vi "skil4.vi"() -> ()   [LabVIEW 2010]
uses:
  <vilib>/Utility/miscctls.llb/LVRectTypeDef.ctl
  lib/Global 2.vi
  <vilib>/Platform/browser.llb/Open URL in Default Browser (path).vi
panel:
  in  "View":bool
  out "Table":string[][](table)
  out "Dev_Gr":cluster{"DevNo":i32, "Group":string}[](array[cluster])
  out "Horizontal:Memory Size":i32 format="%.0p"
  in  "Ed 2":bool
  in  "Ed":bool
  in  "tm":bool
  out "User":string
  out "Device:Temperature":dbl format="%#4.0f"
  out "GPS:Status":i32(ring) items=["Uninitialized", "Antenna Error", "No Useable Satellites", "One Useable Satellite", "Two Useable Satellites", "Three Useable Satellites", "No GPS Time", "PDOP Too High", "Unuseable Satellite", "Fix Rejected", "Self Survey Complete", "Self Survey Not Complete"]
  out "d_h_m_s":dbl caption="в работе (дни, часы, минуты, секунды)" format="%<%D:%H:%M:%S>t"
  out "# elements in queue":i32 caption="Буфер"
  in  "indexhtm":bool
  in  "stop 2":bool
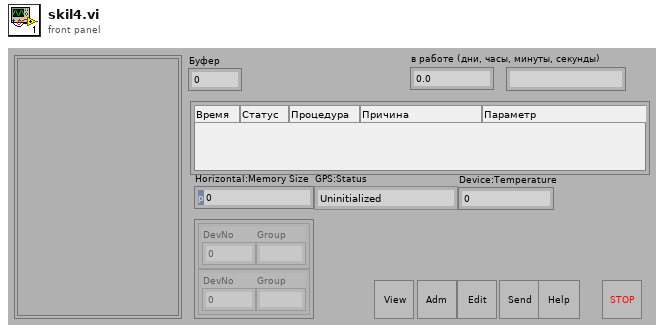
[diagram p1: front panel]
types:
  T1 = cluster{"seconds since 1Jan1904":timestamp, "error out":errorcluster}
  T2 = typedef "LVRectTypeDef.ctl" = cluster{"Left":i16, "Top":i16, "Right":i16, "Bottom":i16}
  T3 = cluster{cluster{"actualSamples":i32, "absoluteInitialX":dbl, "relativeInitialX":dbl, "xIncrement":dbl, "offset":dbl, "gain":dbl, "reserved1":dbl, "reserved2":dbl}[], "wfm":i16[][]}
  T4 = cluster{"Time Stamp":timestamp, "error out":errorcluster}
  T5 = cluster{"adc handle":refnum<k15>, "PN":string, "KR":string}
  T6 = cluster{"seconds since 1Jan1904":timestamp, "error out":errorcluster}[]
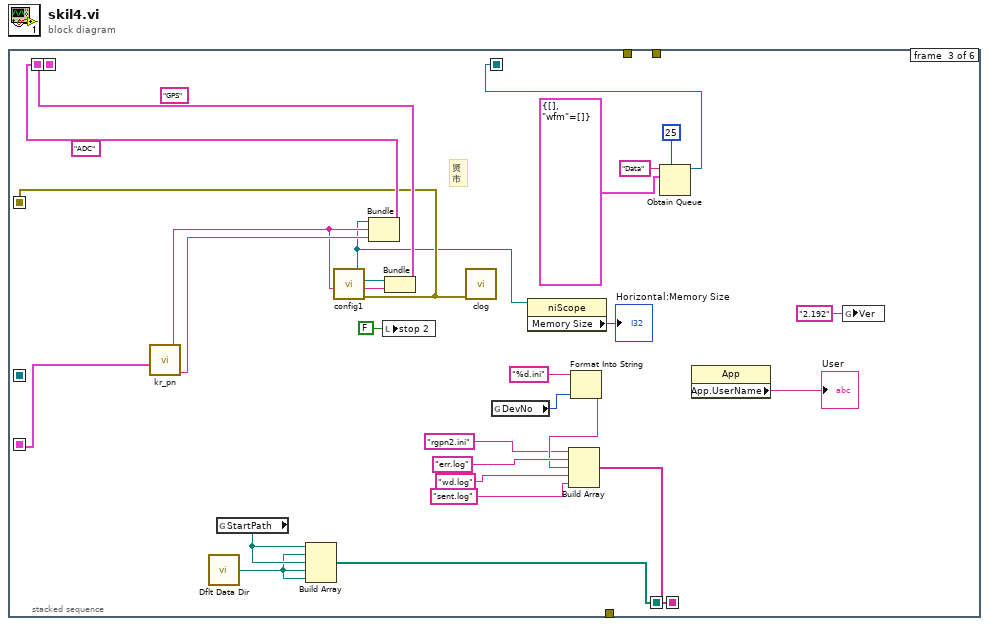
[diagram p0: block diagram]
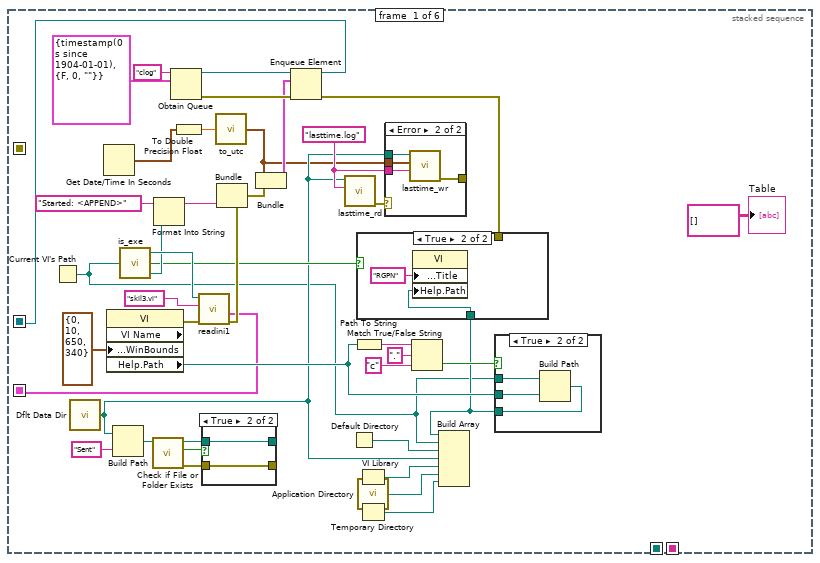
[diagram p2: hidden frame]
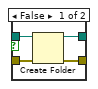
[diagram p6: hidden frame]
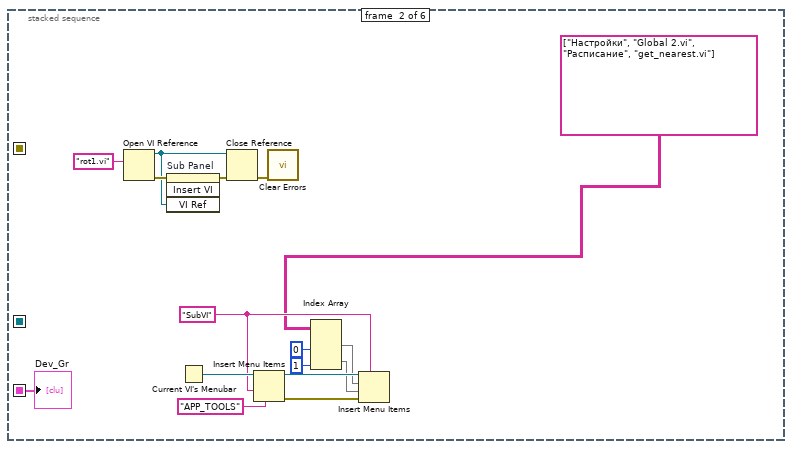
[diagram p7: hidden frame]
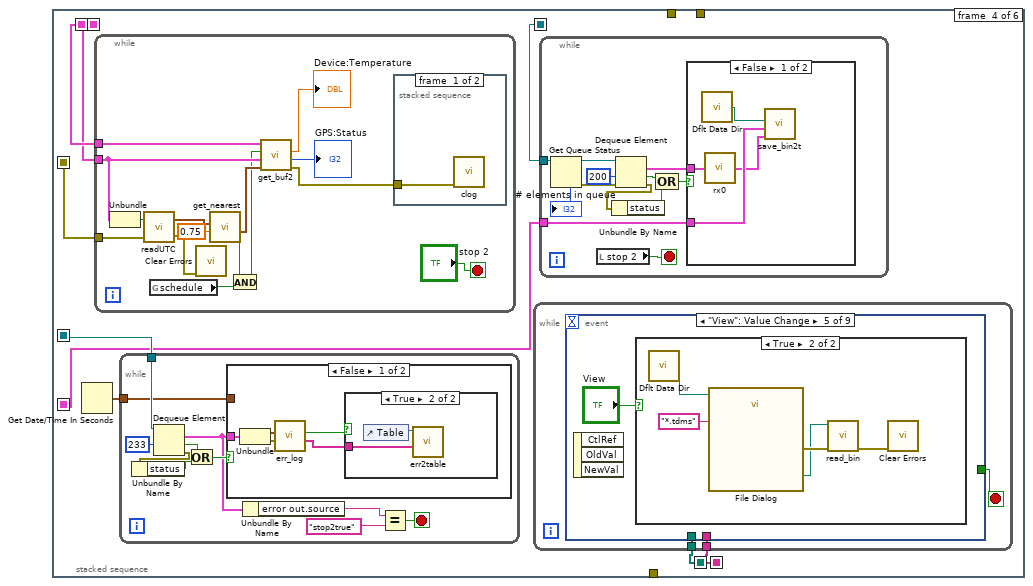
[diagram p8: hidden frame]
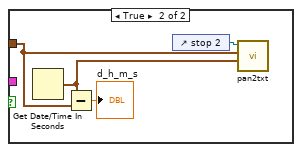
[diagram p10: hidden frame]
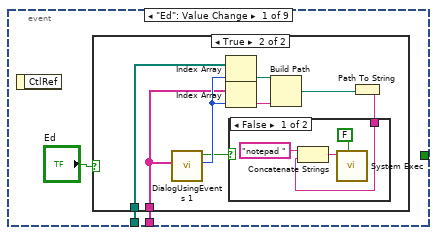
[diagram p11: hidden frame]
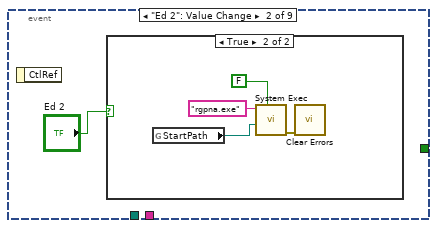
[diagram p14: hidden frame]
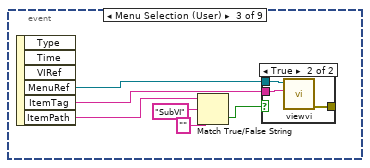
[diagram p16: hidden frame]
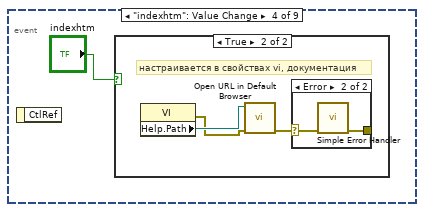
[diagram p18: hidden frame]
diagram:
  n1 = stacked-sequence {
    seq-local: [_ _ w77 _ _ _] -> [_ _ _ w110 w237 _]
    seq-local: [_ _ w101 _ _ _] -> [_ _ _ w109 w243 _]
    seq-local: [_ _ w97 _ _ _] -> [_ _ _ w107 w232 _]
    seq-local: [_ _ w98 _ _ _] -> [_ _ _ w108 w234 _]
    seq-local: [w23 _ _ _ _ _] -> [_ _ _ w106 w228 _]
    seq-local: [_ _ w90 _ _ _] -> [_ _ _ w105 _ _]
    seq-local: [_ _ w89 _ _ _] -> [_ _ _ w104 _ _]
    seq-local: [w6 _ _ _ _ _] -> [_ w71 w82 w102 _ _]
    tunnel: [_ _ _ _ w224 _] -> _
    tunnel: [_ _ _ _ w223 _] -> _
    tunnel: [_ _ _ _ w220 _] -> _
    frame #0 {
      w11 = "lasttime.log" ("name or relative path")
      n2 = Current VI's Path() -> (path=w8:path)
      n3 = call <vilib>:"Dflt Data Dir.vi"() -> ("App:Default Data Directory"=w9:path)
      n4 = Get Date/Time In Seconds() -> (seconds since 1Jan1904=w4:timestamp)
      n5 = property class="VI" props=["VI Name", "Front Panel.WinBounds", "Help.Path"]("Front Panel.WinBounds"=T2 {"Left"=0, "Top"=10, "Right"=650, "Bottom"=340} ("Front Panel Window:Window Bounds")) -> (error out=w40:errorcluster, "Help.Path"=w17:path)  [unwired: 2 in, 2 out]
      n6 = Build Path(base path=w9, name or relative path="Sent") -> (appended path=w37:path)
      n7 = call "is_exe.vi"("path"=w8) -> ("actual path"=w24:path, "exe?"=w22:bool, "ini path"=w41:path)  [unwired: 2 in]
      n8 = call <vilib>:"Check if File or Folder Exists.vi"("path"=w37) -> ("error out"=w34:errorcluster, "file or folder exists?"=w36:bool, "dup path"=w35:path)  [unwired: 8 in]
      n9 = Format Into String(initial string="Started: <APPEND>" ("string"), w24) -> (resulting string=w27:string)  [unwired: 2 in, 1 out]
      n10 = Obtain Queue(name (unnamed)="clog", element data type=T1 {"seconds since 1Jan1904"=timestamp(0 s since 1904-01-01), "error out"={"status"=FALSE, "code"=0, "source"=""}} ("output cluster")) -> (queue out=w31:refnum<queue>, error out=w30:errorcluster)  [unwired: 3 in, 1 out]
      n11 = To Double Precision Float(number=w4) -> (double precision float=w5:dbl)
      n12 = call "readini1.vi"("error in (no error)"=w40, "section"="skil3.vi", "configuration file path"=w41) -> ("error out"=w29:errorcluster, "Dev_Gr"=w6:cluster{"DevNo":i32, "Group":string}[])  [unwired: 1 in, 2 out]
      n13 = case shown="True" w36 {
        tunnel: w35 -> [w55 w57]
        tunnel: w34 -> [w54 w56]
        tunnel: [w53 w57] -> _
        tunnel: [w52 w56] -> _
        frame False {
          n14 = Create Folder(path (use dialog)=w55, error in=w54) -> (created path=w53:path, error out=w52:errorcluster)  [unwired: 1 in, 1 out]
        }
        frame True {
        }
      }
      n15 = call "to_utc.vi"("Numeric"=w5) -> ("Time Stamp"=w3:timestamp)
      n16 = Bundle(cluster=w29, "source"=w27) -> (w26:errorcluster)  [unwired: 2 in]
      n17 = Bundle("Time Stamp"=w3, "error out"=w26) -> (w25:T4)  [unwired: 1 in]
      n18 = Enqueue Element(queue=w31, element=w25, error in (no error)=w30) -> (queue out=w23:refnum<queue>, error out=w21:errorcluster)  [unwired: 1 in, 1 out]
      n19 = call "lasttime_rd.vi"("name or relative path"=w11, "base path"=w9) -> ("error out"=w10:errorcluster)  [unwired: 3 in, 2 out]
      n20 = Default Directory() -> (w18:path)
      n21 = Path To String(path=w17) -> (string=w16:string)
      n22 = VI Library() -> (path=w19:path)
      n23 = call <vilib>:"Application Directory.vi"() -> ("Application Directory"=w7:path)
      n24 = Temporary Directory() -> (w20:path)
      n25 = case shown="Error" w10 {
        tunnel: w3 -> [_ w45]
        tunnel: w11 -> [_ w44]
        tunnel: w9 -> [_ w43]
        tunnel: [_ w42] -> _
        frame No Error {
        }
        frame Error {
          n26 = call "lasttime_wr.vi"("name"=w44, "time stamp"=w45, "start Path"=w43) -> ("error out"=w42:errorcluster)  [unwired: 3 in, 1 out]
        }
      }
      n27 = Match True/False String(2:"c" ("false string"), 3:"." ("true string"), 4:w16) -> (0:w13:bool)  [unwired: 1 out]
      n28 = case shown="True" w13 {
        tunnel: w17 -> [w46 w49]
        tunnel: [w46 w48] -> w12
        tunnel: w8 -> [_ w47]
        frame False {
        }
        frame True {
          n29 = Build Path(base path=w47, name or relative path=w49) -> (appended path=w48:path)
        }
      }
      n30 = case shown="True" w22 {
        tunnel: w21 -> [_ _]
        tunnel: w12 -> [_ w50]
        frame False {
        }
        frame True {
          n31 = property class="VI"("Front Panel.Title"="RGPN" ("Front Panel Window:Title"), "Help.Path"=w50) -> ()  [unwired: 2 in, 2 out]
        }
      }
      n32 = Build Array(w12, w8, w18, w9, w19, w7, w20) -> ()  [unwired: 1 out]
      "Table" <- string[][] [] ("Table")
    }
    frame #1 {
      w59 = "SubVI"
      n33 = Open VI Reference(vi path="rot1.vi") -> (vi reference=w69:refnum<vi>, error out=w72:errorcluster)  [unwired: 5 in]
      n34 = invoke on="Sub Panel" class="SubPanel" method="Insert VI"(error in=w72, "VI Ref"=w69) -> (error out=w70:errorcluster)  [unwired: 2 in, 3 out]
      n35 = Current VI's Menubar() -> (w67:refnum<k9>)
      n36 = Close Reference(reference=w69, error in (no error)=w70) -> (error out=w68:errorcluster)
      n37 = Insert Menu Items(4:"APP_TOOLS" ("after item"), 7:w59, 9:w67) -> (0:w65:errorcluster, 3:w66:refnum<k9>)  [unwired: 3 in, 1 out]
      n38 = call <vilib>:"Clear Errors.vi"("error in (no error)"=w68) -> ()  [unwired: 6 in, 1 out]
      n39 = Index Array(array=string[][] [["Настройки", "Global 2.vi"], ["Расписание", "get_nearest.vi"]], index (col) #1=0 ("disabled index (col)"), index (col) #2=1 ("index (col)")) -> (element #1=w63:string[], element #2=w62:string[])  [unwired: 2 in]
      n40 = Insert Menu Items(5:w59, 6:w65, 7:w62, 8:w63, 9:w66) -> ()  [unwired: 1 in, 3 out]
      "Dev_Gr" <- w71
    }
    frame #2 {
      (unwired) "GPS"
      (unwired) "ADC"
      # "贤\n市"
      n41 = call "kr_pn.vi"("Dev_Gr"=w82) -> ("KR"=w84:string, "PN"=w83:string)  [unwired: 3 in, 2 out]
      n42 = call <vilib>:"Dflt Data Dir.vi"() -> ("App:Default Data Directory"=w78:path)
      n43 = global read "Global 2.vi" "StartPath"() -> (w87:path)
      n44 = Build Array(w87, w78, w87, w78, w78) -> (w90:path[])
      n45 = call "config1.vi"("ChList"=w83) -> ("error out"=w77:errorcluster, "trig"=w99:tag, "gps handle"=w100:refnum<k15>, "adc handle"=w76:refnum<k15>)  [unwired: 3 in]
      n46 = Bundle("adc handle"=w76, "PN"=w83, "KR"=w84) -> (w98:T5)  [unwired: 1 in]
      n47 = local write "stop 2"(FALSE ("stop 2")) -> ()
      n48 = Bundle("gps handle"=w100, "trig"=w99) -> (w97:cluster{"gps handle":refnum<k15>, "trig":tag})  [unwired: 1 in]
      n49 = call "clog.vi"("error"=w77) -> ()  [unwired: 7 in]
      n50 = global read "Global 2.vi" "DevNo"() -> (w86:i32)
      n51 = property class="niScope"(reference=w76) -> ("Memory Size"=→"Horizontal:Memory Size":i32)  [unwired: 1 in, 2 out]
      n52 = Format Into String(format string="%d.ini", w86) -> (resulting string=w91:string)  [unwired: 2 in, 1 out]
      n53 = Build Array("rgpn2.ini" ("element"), "err.log", w91, "wd.log", "sent.log") -> (w89:string[])
      n54 = Obtain Queue(max queue size (-1, unlimited)=25, name (unnamed)="Data", element data type=T3 {[], "wfm"=[]} ("Cluster")) -> (queue out=w101:refnum<queue>)  [unwired: 2 in, 2 out]
      n55 = property class="App"() -> ("App.UserName"=→"User":string)  [unwired: 2 in, 2 out]
      n56 = global write "Global 2.vi" "Ver"("2.192" ("Ver")) -> ()
    }
    frame #3 {
      n57 = Get Date/Time In Seconds() -> (seconds since 1Jan1904=w103:timestamp)
      n58 = while {
        tunnel: w110 -> [w208]
        tunnel: w107 -> [w215]
        tunnel: w108 -> [w213]
        stop <- "stop 2" stop-if-true
        n59 = Unbundle(w215) -> ("gps handle"=w214:refnum<k15>)  [unwired: 1 out]
        n60 = call "readUTC.vi"("error out 2"=w208, "gps handle"=w214) -> ("error out"=w204:errorcluster, "time"=w216:timestamp)
        n61 = global read "Global 2.vi" "schedule"() -> (w205:bool)
        n62 = call <vilib>:"Clear Errors.vi"("error in (no error)"=w204) -> ()  [unwired: 6 in, 1 out]
        n63 = call "get_nearest.vi"("interval_sec"=0.75, "current time"=w216) -> ("found"=w207:bool, "next_TimeStamp"=w211:timestamp)  [unwired: 3 in, 1 out]
        n64 = And(x=w207, y=w205) -> (x .and. y?=w206:bool)
        n65 = call "get_buf2.vi"("time GPS"=w211, "Sync cluster"=w215, "Boolean"=w206, "Scope Cluster"=w213) -> ("error out"=w202:errorcluster, "Timing:GPS:Status"=→"GPS:Status":i32, "Device:Temperature"=→"Device:Temperature":dbl)  [unwired: 1 in]
        n66 = stacked-sequence {
          tunnel: w202 -> [w217 w219]
          frame #0 {
            n67 = call "clog.vi"("error"=w217) -> ()  [unwired: 7 in]
          }
          frame #1 {
            n68 = control-ref of="stop 2"() -> (w218:refnum<vi>)
            n69 = call "restart1.vi"("error in"=w219, "Bool Refnum"=w218) -> ()
          }
        }
      }
      n70 = while {
        tunnel: w106 -> [w120]
        tunnel: w103 -> [w115]
        stop <- w113 stop-if-true
        n71 = Dequeue Element(queue=w120, timeout in ms (-1)=233) -> (element=w112:T1, timed out?=w117:bool, error out=w119:errorcluster)  [unwired: 1 in, 1 out]
        n72 = Unbundle By Name(w119) -> ("status"=w118:bool)
        n73 = Or(x=w117, y=w118) -> (x .or. y?=w116:bool)
        n74 = case shown="False" w116 {
          tunnel: w112 -> [w124 _]
          tunnel: w115 -> [_ w130]
          frame False {
            n75 = Unbundle(w124) -> ("seconds since 1Jan1904"=w126:timestamp, "error out"=w125:errorcluster)
            n76 = call "err_log.vi"("error In"=w125, "time stamp"=w126) -> ("err_table"=w123:string[], "do?"=w122:bool)  [unwired: 4 in]
            n77 = case shown="True" w122 {
              tunnel: w123 -> [_ w127]
              frame False {
              }
              frame True {
                n78 = control-ref of="Table"() -> (w128:refnum<vi>)
                n79 = call "err2table.vi"("err_table"=w127, "Tbl Refnum"=w128) -> ()  [unwired: 6 in]
              }
            }
          }
          frame True {
            n80 = Get Date/Time In Seconds() -> (seconds since 1Jan1904=w131:timestamp)
            n81 = Subtract(x=w131, y=w130) -> (x-y=→"d_h_m_s":dbl)
            n82 = control-ref of="stop 2"() -> (w129:refnum<vi>)
            n83 = call "pan2txt.vi"("seconds since 1Jan1904"=w131, "started"=w130, "stop button"=w129) -> ()  [unwired: 5 in]
          }
        }
        n84 = Unbundle By Name(w112) -> ("error out.source"=w111:string)
        n85 = Equal?(x=w111, y="stop2true" ("source")) -> (x = y?=w113:bool)
      }
      n86 = while {
        tunnel: w105 -> [w134]
        tunnel: w104 -> [w133]
        stop <- w135 stop-if-true
        n87 = event shown="[4] \"View\": Value Change" {
          selector: _ -> [_ _ _ _ _ _ _ _ _]
          dyn-events: _ -> [_ _ _ _ _ _ _ _ _]
          timeout: _ -> [_ _ _ _ _ _ _ _ _]
          tunnel: [_ _ _ _ _ _ w182 _ _] -> w135
          tunnel: w134 -> [w137 _ _ _ _ _ _ _ _]
          tunnel: w133 -> [w136 _ _ _ _ _ _ _ _]
          event "Ed": Value Change {
            n88 = event-data() -> ()  [unwired: 1 in, 1 out]
            n89 = case shown="True" "Ed" {
              tunnel: w137 -> [_ w140]
              tunnel: w136 -> [_ w139]
              frame False {
              }
              frame True {
                n90 = call "DialogUsingEvents 1.vi"("Strings []"=w139) -> ("Numeric"=w146:i32, "Cancelled?"=w141:bool)  [unwired: 8 in, 1 out]
                n91 = Index Array(array=w140, index=w146) -> (element=w145:path)
                n92 = Index Array(array=w139, index=w146) -> (element=w144:string)
                n93 = Build Path(base path=w145, name or relative path=w144) -> (appended path=w143:path)
                n94 = Path To String(path=w143) -> (string=w142:string)
                n95 = case shown="False" w141 {
                  tunnel: w142 -> [w149 _]
                  frame False {
                    n96 = Concatenate Strings("notepad " ("string"), w149) -> (w148:string)
                    n97 = call <vilib>:"System Exec.vi"("wait until completion? (T)"=FALSE, "command line"=w148) -> ()  [unwired: 6 in, 4 out]
                  }
                  frame True {
                  }
                }
              }
            }
          }
          event "Ed 2": Value Change {
            n98 = event-data() -> ()  [unwired: 1 in, 1 out]
            n99 = case shown="True" "Ed 2" {
              frame False {
              }
              frame True {
                n100 = global read "Global 2.vi" "StartPath"() -> (w154:path)
                n101 = call <vilib>:"System Exec.vi"("wait until completion? (T)"=FALSE, "working directory"=w154, "command line"="rgpna.exe") -> ("error out"=w152:errorcluster)  [unwired: 5 in, 3 out]
                n102 = call <vilib>:"Clear Errors.vi"("error in (no error)"=w152) -> ()  [unwired: 6 in, 1 out]
              }
            }
          }
          event Menu Selection (User) {
            n103 = event-data() -> ("MenuRef"=w159:refnum<k9>, "ItemTag"=w158:string, "ItemPath"=w157:string)  [unwired: 1 in, 3 out]
            n104 = Match True/False String(2:"" ("false string"), 3:"SubVI" ("true string"), 4:w157) -> (0:w160:bool)  [unwired: 1 out]
            n105 = case shown="True" w160 {
              tunnel: w159 -> [_ w164]
              tunnel: [_ w163] -> _
              tunnel: w158 -> [_ w162]
              frame False {
              }
              frame True {
                n106 = call "viewvi.vi"("item tag"=w162, "menu reference"=w164) -> ("error out"=w163:errorcluster)  [unwired: 5 in]
              }
            }
          }
          event "indexhtm": Value Change {
            n107 = event-data() -> ()  [unwired: 1 in, 1 out]
            n108 = case shown="True" "indexhtm" {
              frame False {
              }
              frame True {
                # "настраивается в свойствах vi, документация"
                n109 = property class="VI"() -> (error out=w166:errorcluster, "Help.Path"=w167:path)  [unwired: 2 in, 1 out]
                n110 = call-poly <vilib>:"Open URL in Default Browser.vi"("error in (no error)"=w166, "path"=w167) -> ("error out"=w168:errorcluster)  [unwired: 4 in, 1 out]
                n111 = case shown="Error" w168 {
                  selector: w168 -> [_ w170]
                  tunnel: [_ w169] -> _
                  frame No Error {
                  }
                  frame Error {
                    n112 = call <vilib>:"Simple Error Handler.vi"("error in (no error)"=w170) -> ("error out"=w169:errorcluster)  [unwired: 4 in, 4 out]
                  }
                }
              }
            }
          }
          event "View": Value Change {
            n113 = event-data() -> ()  [unwired: 1 in, 3 out]
            n114 = case shown="True" "View" {
              frame False {
              }
              frame True {
                n115 = call <vilib>:"Dflt Data Dir.vi"() -> ("App:Default Data Directory"=w176:path)
                n116 = call "File Dialog"("start path"=w176, "pattern (all files)"="*.tdms") -> ("selected path"=w174:path, "error out"=w175:errorcluster)  [unwired: 10 in, 2 out]
                n117 = call "read_bin.vi"("error in"=w175, "datalog path"=w174) -> ("error out"=w173:errorcluster)  [unwired: 2 in, 3 out]
                n118 = call <vilib>:"Clear Errors.vi"("error in (no error)"=w173) -> ()  [unwired: 6 in, 1 out]
              }
            }
          }
          event "tm": Value Change {
            n119 = event-data() -> ()  [unwired: 1 in, 1 out]
            n120 = case shown="True" "tm" {
              tunnel: [_ w179] -> _
              frame False {
              }
              frame True {
                n121 = global read "Global 2.vi" "StartPath"() -> (w178:path)
                n122 = call <vilib>:"System Exec.vi"("wait until completion? (T)"=FALSE, "working directory"=w178, "command line"="skil2.exe") -> ("error out"=w179:errorcluster)  [unwired: 5 in, 3 out]
              }
            }
          }
          event "stop 2": Value Change {
            n123 = event-data() -> ("NewVal"=w182:bool)  [unwired: 1 in, 4 out]
            n124 = case shown="True" w182 {
              frame False {
              }
              frame True {
                n125 = call "clog.vi"("error"=errorcluster {"status"=TRUE, "code"=0, "source"="stop2true"}) -> ()  [unwired: 7 in]
              }
            }
          }
          event Application Instance Close? {
            w184 = TRUE ("Value (Signaling)")
            n126 = event-data() -> ()  [unwired: 1 in, 4 out]
            n127 = property on="stop 2" class="Bool (strict)"("Val(Sgnl)"=w184) -> ()  [unwired: 2 in, 2 out]
            n128 = event-data("Discard?"=w184) -> ()  [unwired: 2 in, 1 out]
          }
          event Panel Close? {
            w185 = TRUE ("Value (Signaling)")
            n129 = event-data() -> ()  [unwired: 1 in, 3 out]
            n130 = property on="stop 2" class="Bool (strict)"("Val(Sgnl)"=w185) -> ()  [unwired: 2 in, 2 out]
            n131 = event-data("Discard?"=w185) -> ()  [unwired: 1 in, 1 out]
          }
        }
      }
      n132 = while {
        tunnel: w109 -> [w196]
        tunnel: w102 -> [w187]
        stop <- w186 stop-if-true
        n133 = Get Queue Status(queue=w196) -> (queue out=w195:refnum<queue>, error out=w194:errorcluster, # elements in queue=→"# elements in queue":i32)  [unwired: 2 in, 5 out]
        n134 = local read "stop 2"() -> (w186:bool)
        n135 = Dequeue Element(queue=w195, timeout in ms (-1)=200, error in (no error)=w194) -> (element=w188:T3, timed out?=w191:bool, error out=w192:errorcluster)  [unwired: 1 out]
        n136 = Unbundle By Name(w192) -> ("status"=w190:bool)
        n137 = Compound Arithmetic op=OR(w191, w190) -> (w189:bool)
        n138 = case shown="False" w189 {
          tunnel: w188 -> [w199 _]
          tunnel: w187 -> [w200 _]
          frame False {
            n139 = call <vilib>:"Dflt Data Dir.vi"() -> ("App:Default Data Directory"=w201:path)
            n140 = call "rx0.vi"("Cluster 2"=w199) -> ("Cluster"=w198:T3)
            n141 = call "save_bin2t.vi"("Cluster"=w198, "Dev_Gr"=w200, "Data Directory"=w201) -> ()  [unwired: 1 in]
          }
          frame True {
          }
        }
      }
    }
    frame #4 {
      n142 = Unbundle(w234) -> ("adc handle"=w233:refnum<k15>)  [unwired: 2 out]
      n143 = call <instrlib>:"niScope Abort.vi"("instrument handle"=w233, "error in"=w237) -> ("instrument handle out"=w245:refnum<k15>, "error out"=w244:errorcluster)  [unwired: 12 in]
      n144 = call <instrlib>:"niScope Close.vi"("instrument handle"=w245, "error in"=w244) -> ("error out"=w238:errorcluster)  [unwired: 13 in]
      n145 = Get Queue Status(queue=w228, return elements? (F)=TRUE) -> (queue out=w226:refnum<queue>, error out=w221:errorcluster, elements=w225:T6)  [unwired: 1 in, 5 out]
      n146 = for {
        tunnel: w225 -> [w248] mode=indexing
        n147 = Unbundle(w248) -> ("seconds since 1Jan1904"=w247:timestamp, "error out"=w246:errorcluster)
        n148 = call "err_log.vi"("error In"=w246, "time stamp"=w247) -> ()  [unwired: 4 in, 2 out]
      }
      n149 = Unbundle(w232) -> ("gps handle"=w231:refnum<k15>, "trig"=w230:tag)
      n150 = call <instrlib>:"niSync Disable Time Stamp Trigger.vi"("error in (no error)"=w238, "terminal"=w230, "instrument handle"=w231) -> ("error out"=w241:errorcluster, "instrument handle out"=w242:refnum<k15>)  [unwired: 6 in]
      n151 = call <instrlib>:"niSync Disconnect Trigger Terminals.vi"("error in (no error)"=w241, "destination terminal"="AllConnected", "source terminal"="AllConnected", "instrument handle"=w242) -> ("error out"=w240:errorcluster, "instrument handle out"=w239:refnum<k15>)  [unwired: 6 in]
      n152 = Release Queue(queue=w226, force destroy? (F)=TRUE, error in (no error)=w221) -> (error out=w220:errorcluster)  [unwired: 2 out]
      n153 = Release Queue(queue=w243, force destroy? (F)=TRUE) -> (error out=w223:errorcluster)  [unwired: 1 in, 2 out]
      n154 = call <instrlib>:"niSync Close.vi"("error in (no error)"=w240, "instrument handle"=w239) -> ("error out"=w224:errorcluster)  [unwired: 9 in]
    }
    frame #5 {
      n155 = Current VI's Path() -> (path=w252:path)
      n156 = call "is_exe.vi"("path"=w252) -> ("exe?"=w251:bool)  [unwired: 2 in, 2 out]
      n157 = Not(x=w251) -> (.not. x?=w250:bool)
      n158 = Quit LabVIEW(quit? (T)=w251) -> ()
      n159 = Request Deallocation(w250) -> ()
      n160 = local write "stop 2"(FALSE ("stop 2")) -> ()
    }
  }
